vi "CAN test do RIO 2.vi"() -> ()   [LabVIEW 2014]
doc: "This example demonstrates frame streaming output using an NI-Embedded CAN for RIO interface. \n\nThis example can run against any input example, assuming you have a properly terminated CAN cable connected to two CAN ports."
uses:
  <vilib>/RioEmbeddedCAN/RioEmbeddedCAN.llb/CANFrameControl.ctl
  <vilib>/Platform/TimedLoop/XDataNode/timing_clust.ctl
  <vilib>/Platform/TimedLoop/XDataNode/nitl_modes.ctl
  <vilib>/Platform/TimedLoop/XDataNode/wakeup.ctl
  <vilib>/Platform/TimedLoop/XDataNode/XDataNode.xnode
  <vilib>/Platform/TimedLoop/XDataNode/XDNodeRunTimeDep.lvlib
  <resource>/objmgr/RioEmbeddedCANInterface.rc
  <vilib>/Utility/Variable/NI_VariableUtilities.lvlib
  Data Communication/Network Streams/Simple Network Streams/support/Network Stream Command.ctl
  <vilib>/RioEmbeddedCAN/RioEmbeddedCAN.llb/CANWaitTransmitComplete.vi
panel:
  out "okres":dbl
  out "value":T1 {"type" items=["CAN Data", "CAN Remote"]; "identifier" format="%.0x"}
  in  "stop 3":bool
  out "ilosc mesag 2":dbl
  out "Frames 3":string[][](table) caption="Frames"
  out "Numeric 2":i32
  in  "Number of Frames to Display 3":i32=15
  in  "stop 5":bool
  out "data string":string
  in  "stop 4":bool
  out "appended array":string[](array[string])
  out "ilosc mesag":dbl
  out "Numeric":i32
  in  "stop 2":bool
  out "Waveform Chart 5":cluster{"mean":dbl, "output 3":u16}(graph)
  out "Waveform Chart 2":cluster{"rms value":dbl, "output 2":dbl}(graph)
  in  "odczyt 2":bool=TRUE
  out "Frames 2":string[][](table) caption="Frames"
  in  "Number of Frames to Display 2":i32=15
  in  "Hexadecimal? 2":bool
  out "error out":errorcluster
  out "x != y?":bool
  out "(hi.lo)":u16
  out "x .or. y?":bool
  out "data":T1[](array[typedef]) {"type" items=["CAN Data", "CAN Remote"]; "identifier" format="%.0x"}
  in  "stop":bool
  out "Variable2":bool
  in  "CAN frame 2":T1={"identifier"=2, "extended?"=FALSE, "type"=0, "payload"=[1, 2, 3, 4, 5, 6, 7, 8]} {"type" items=["CAN Data", "CAN Remote"]; "identifier" format="%.0x"}
  in  "Stop Button":bool
  in  "Write":bool
  in  "CAN frame":T1={"identifier"=2, "extended?"=FALSE, "type"=0, "payload"=[1, 2, 3, 4, 5, 6, 7, 8]} {"type" items=["CAN Data", "CAN Remote"]; "identifier" format="%.0x"}
  in  "receive queue size":u32=50
  in  "baud rate":u32=500000
  in  "interface index":u32
  # "Overview: Demonstrates frame streaming output using an NI-Embedded CAN for RIO interface.\nInstructions: Run the VI."
  # "See VI Info <Ctrl+I> for more information on how to use this example"
  # "Interface Configuration"
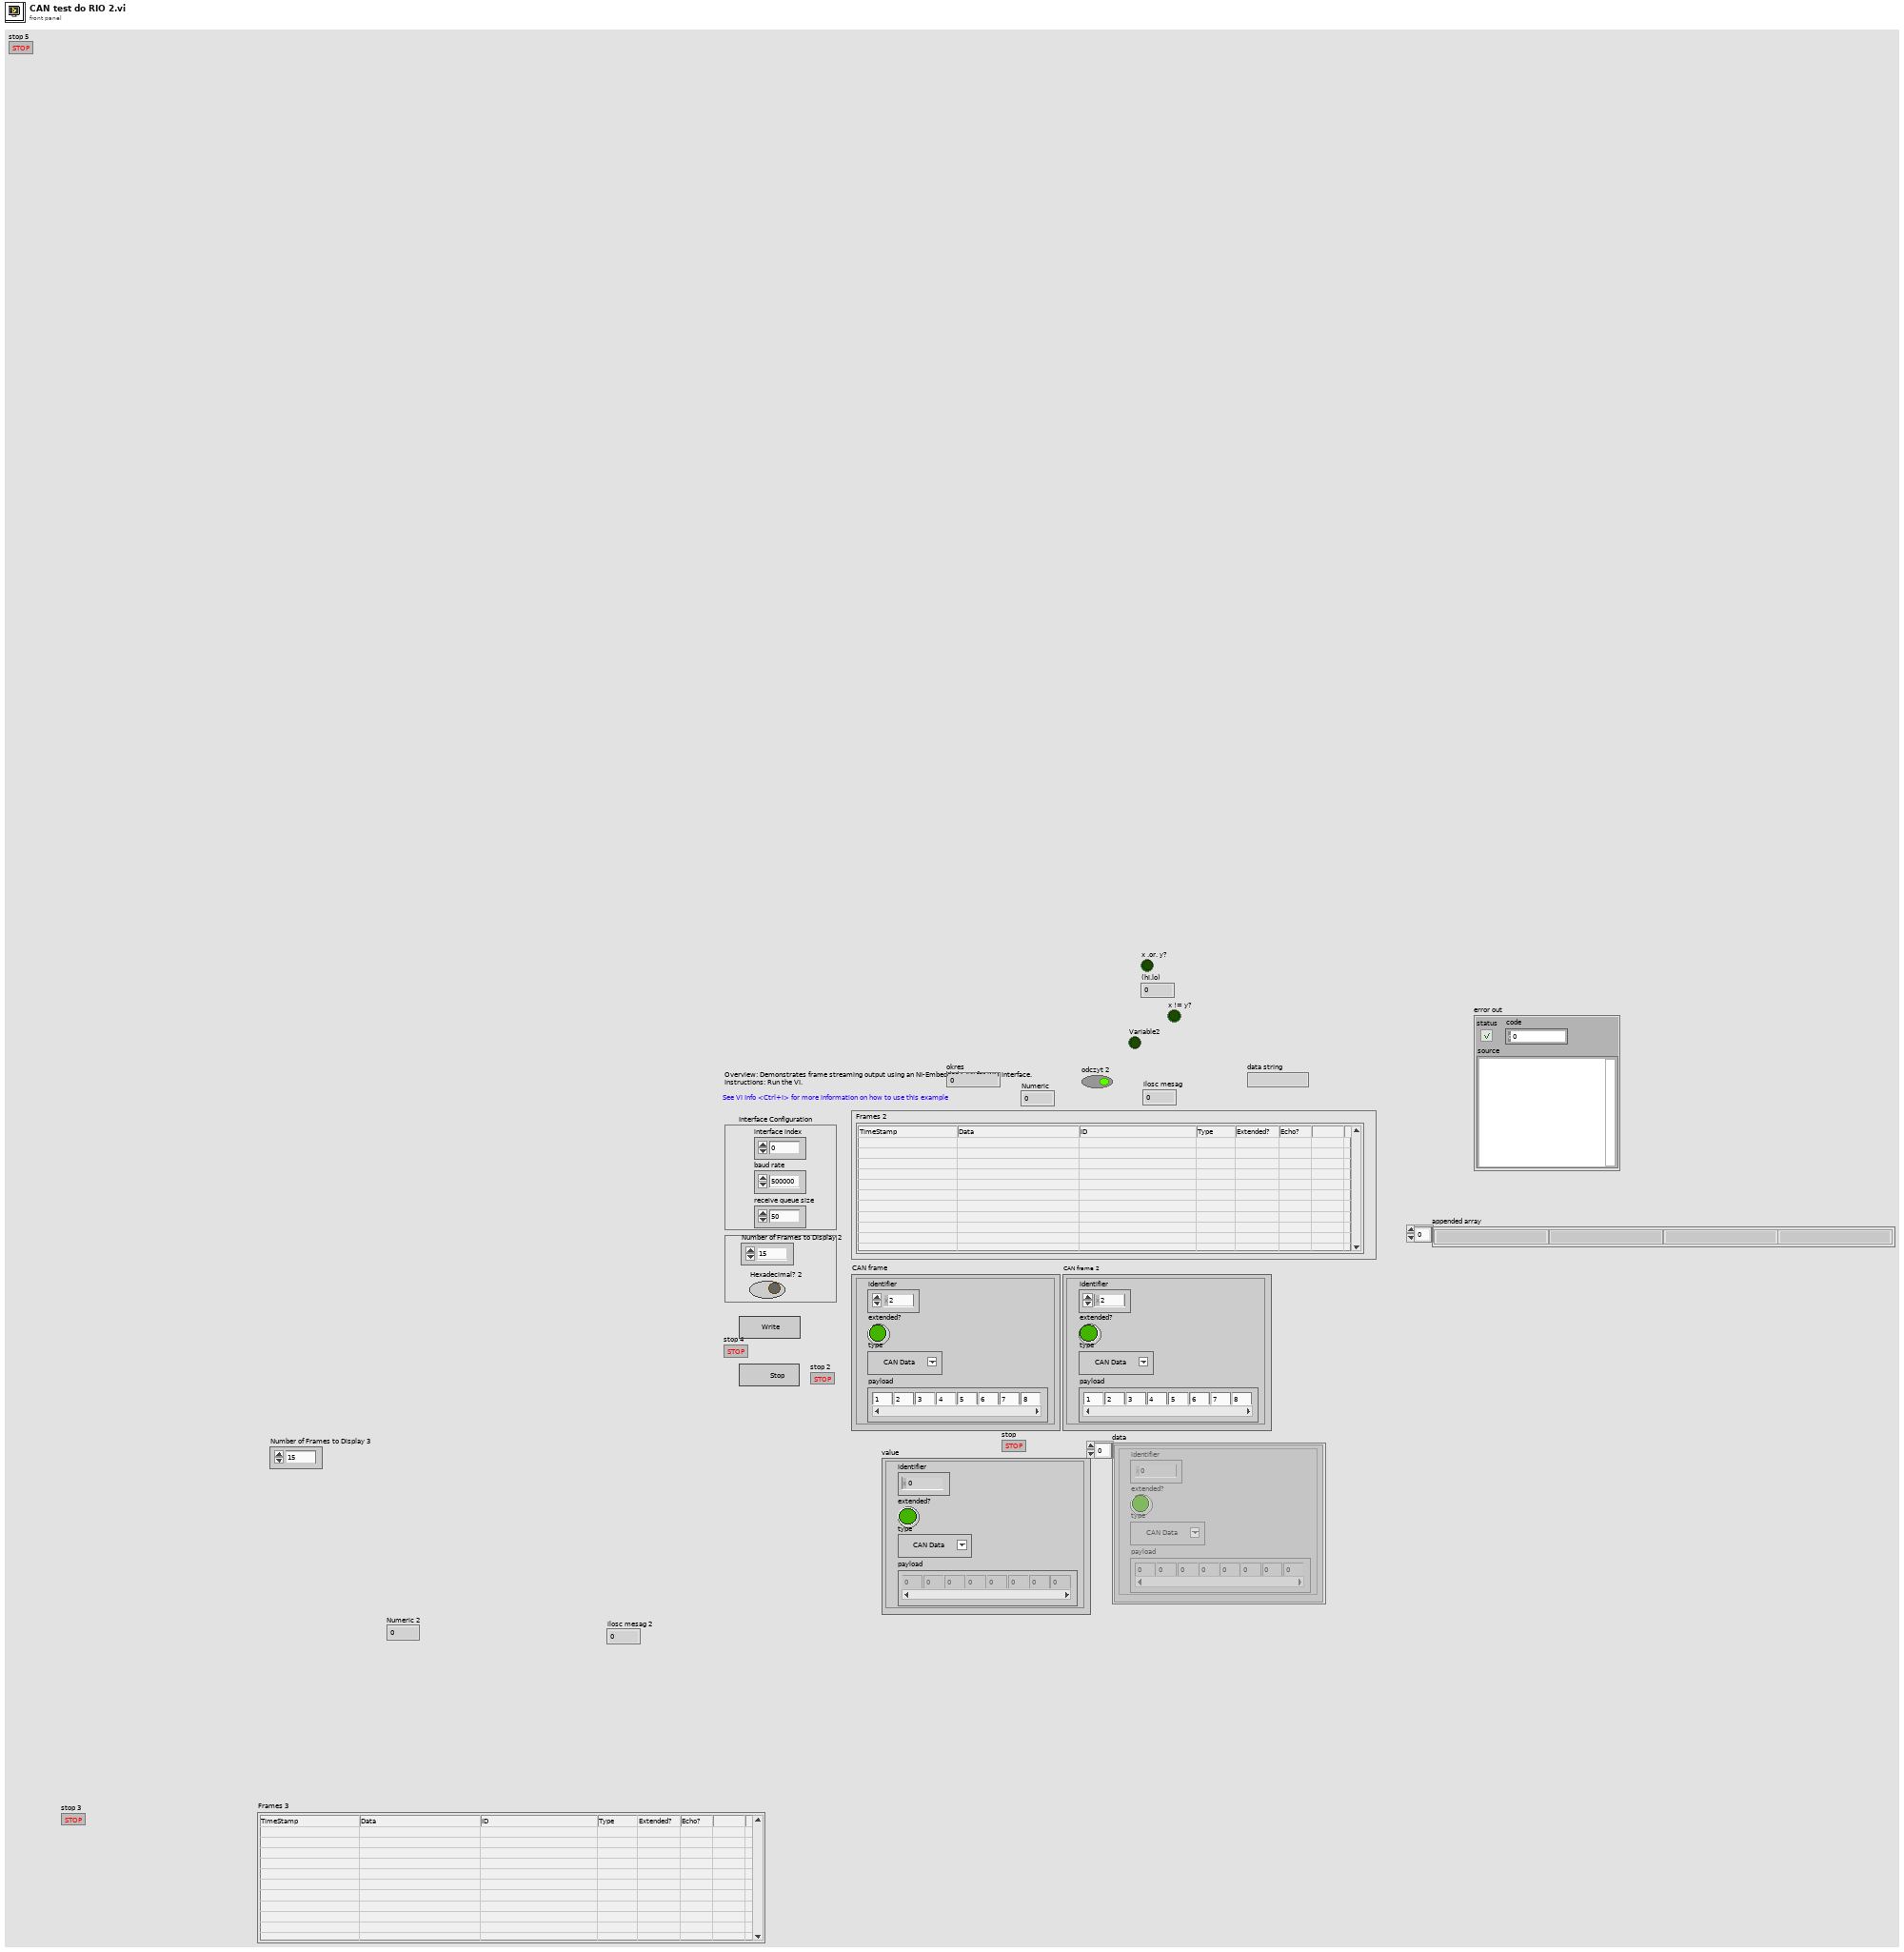
[diagram p1: front panel]
types:
  T1 = typedef "CANFrameControl.ctl" = cluster{"identifier":u32, "extended?":bool, "type":u8, "payload":u8[]}
  T2 = typedef "XDNodeRunTimeDep.lvlib/timing_clust.ctl" = cluster{"Expected End [f-1]":u64, "Actual End [f-1]":u64, "Finished Late? [f-1]":bool, "Expected End [i-1]":u64, "Actual End [i-1]":u64, "Finished Late? [i-1]":bool, "Expected Start [i]":u64, "Actual Start [i]":u64, "Expected Start [f]":u64, "Actual Start [f]":u64, "Source Name":string, "Structure Name":string, "Period":i64, "Deadline":i64, "Offset":i64, "Start":i64, "Priority":i32, "Timeout":i32, "Mode":T3, "Wakeup Reason":T4, "Error":errorcluster, "Source Type":string, "Secondary Source Type":string, "Global End Time":u64, "Global Start Time":u64, "Frame Duration":u64, "Iteration Duration":u64, "Assigned CPU":i32, "I/O Scan Engine Mode":u32}
  T3 = typedef "XDNodeRunTimeDep.lvlib/nitl_modes.ctl" = enum32{"No Change", "Process missed periods, maintain original phase", "Discard missed periods, maintain original phase", "Process missed periods, ignore original phase", "Discard missed periods, ignore original phase"}
  T4 = typedef "XDNodeRunTimeDep.lvlib/wakeup.ctl" = enum32{"Normal", "Aborted", "Asynchronous wakeup", "Timing source error", "Timed loop error", "Timeout"}
  T5 = typedef "Network Stream Command.ctl" = cluster{"Message":string, "Message Data":variant}
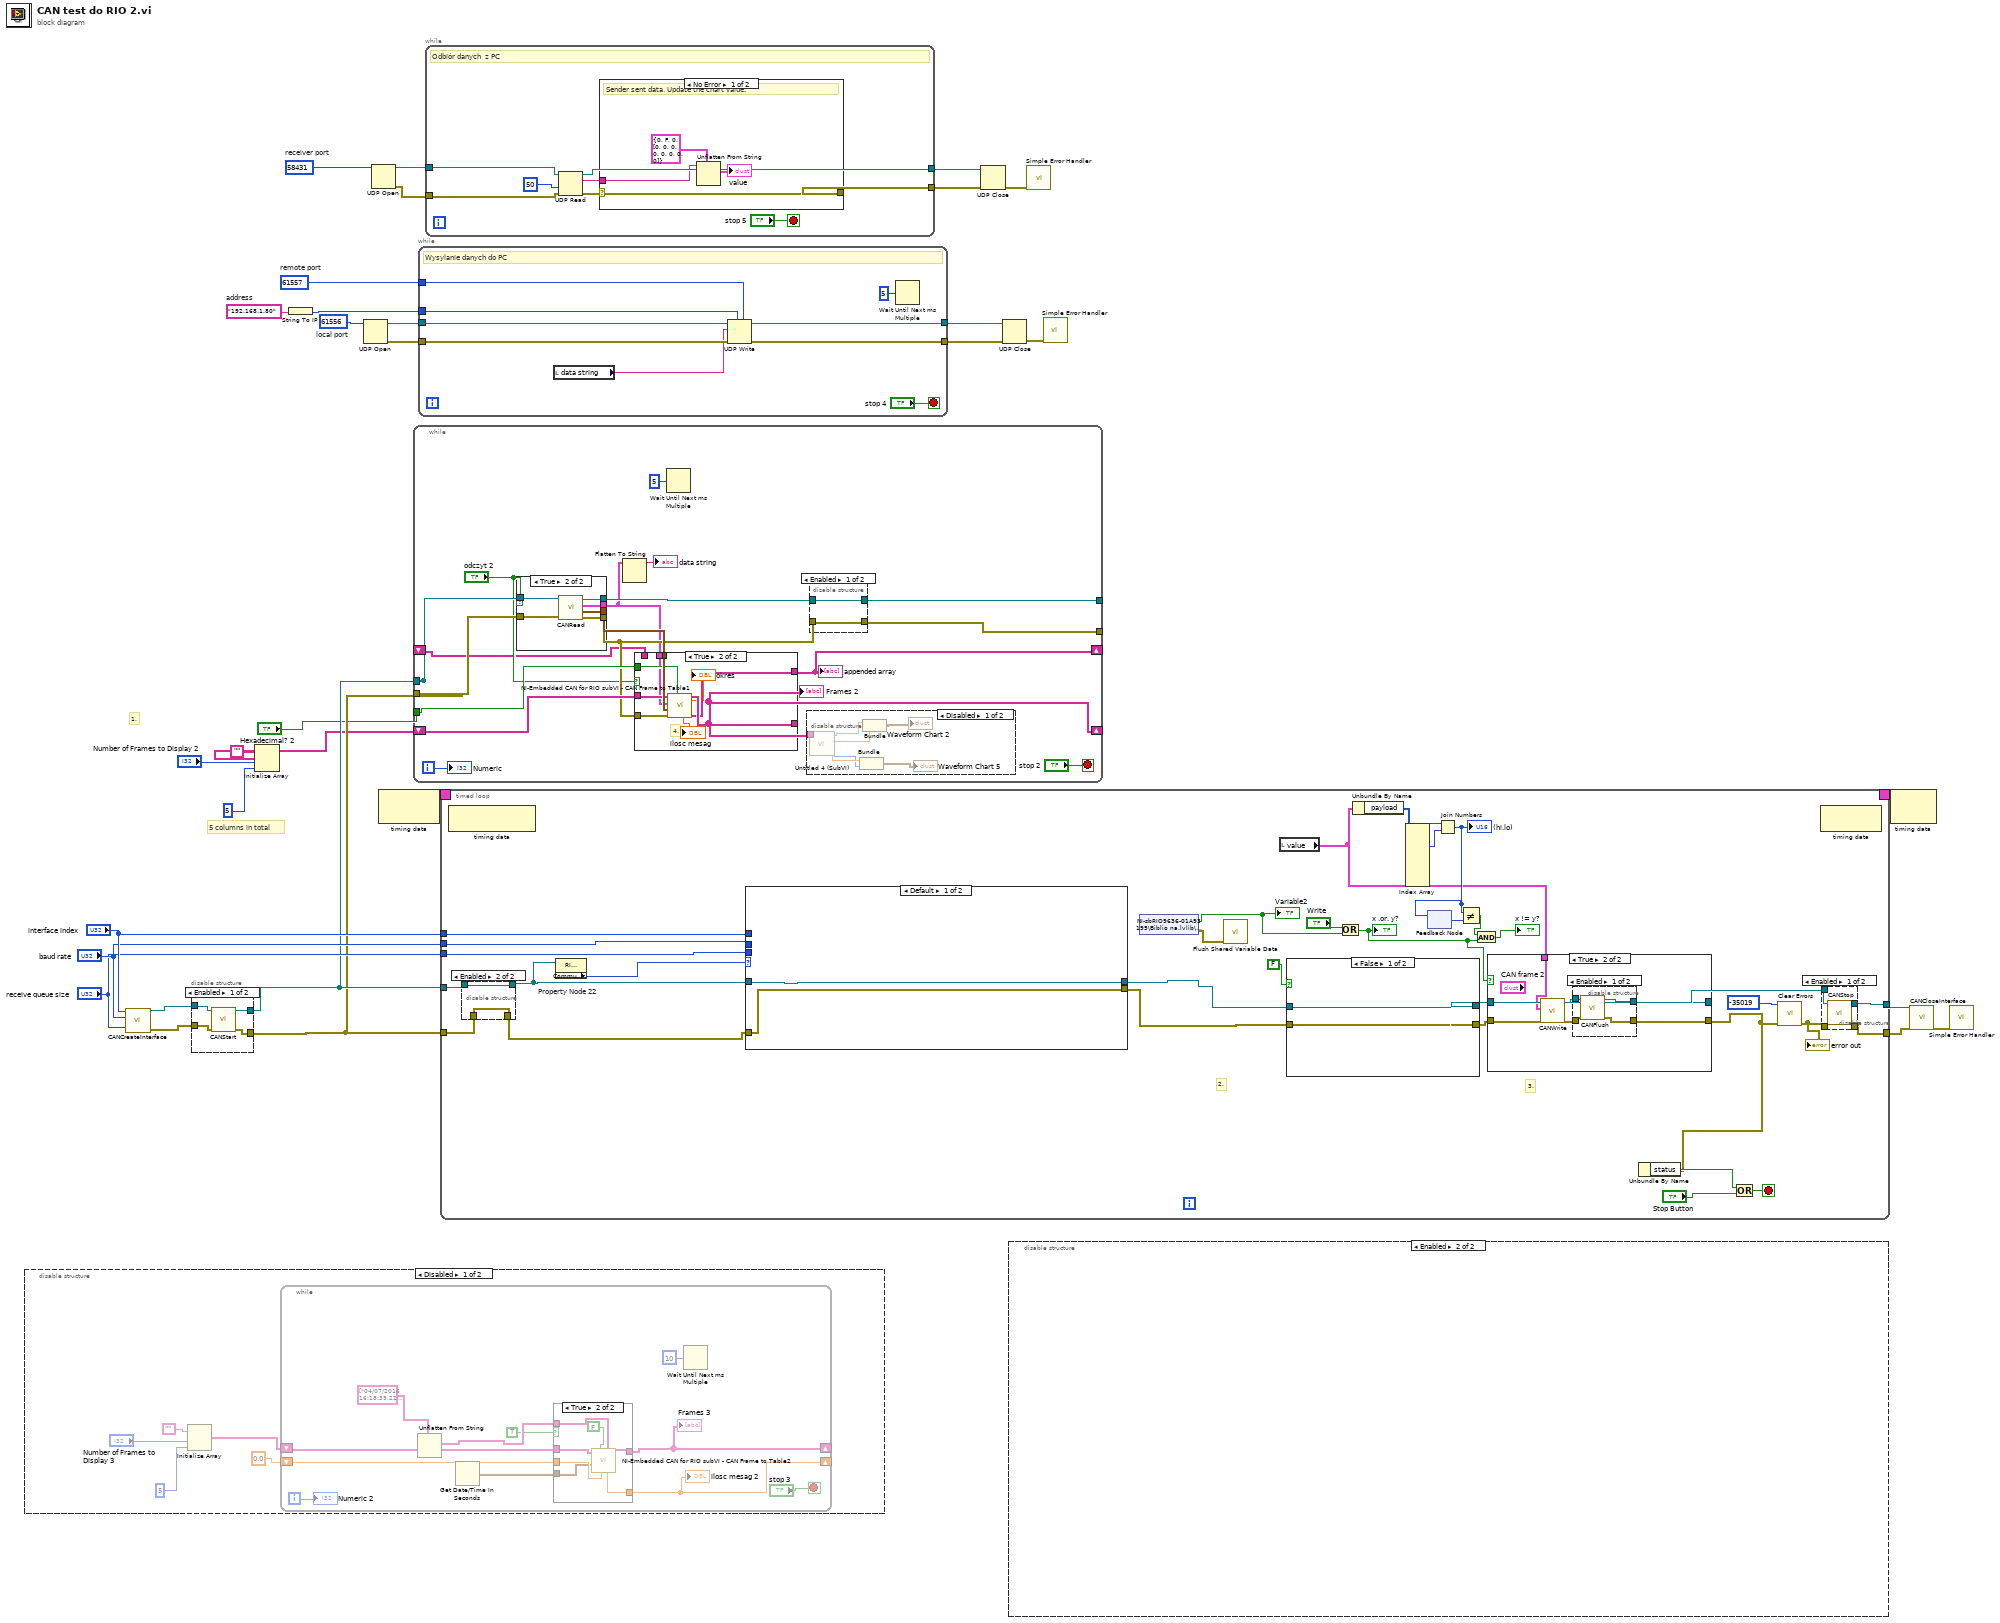
[diagram p0: block diagram]
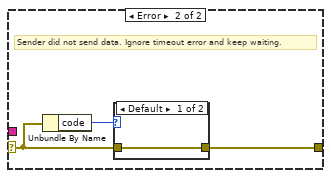
[diagram p4: hidden frame]
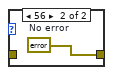
[diagram p5: hidden frame]
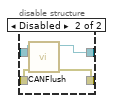
[diagram p8: hidden frame]
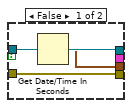
[diagram p9: hidden frame]
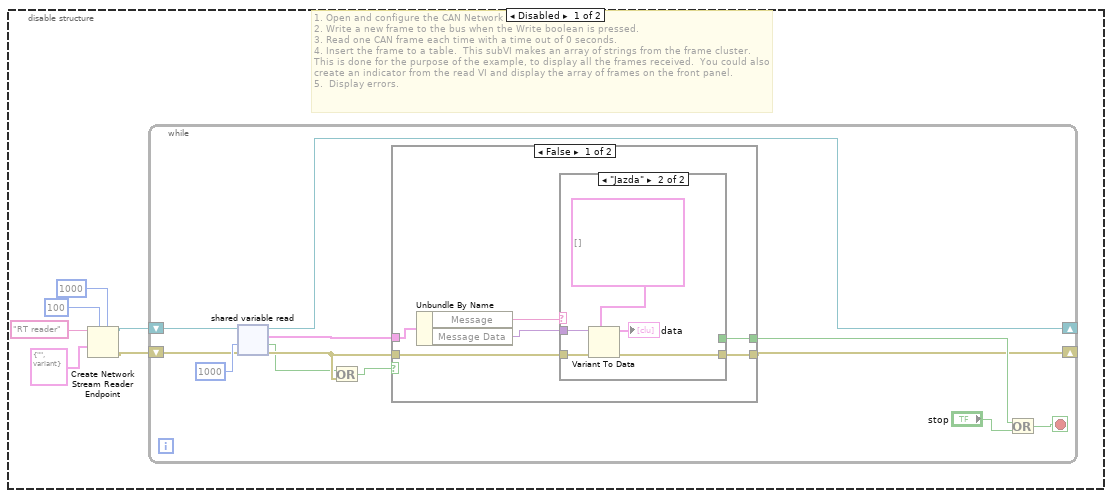
[diagram p11: hidden frame]
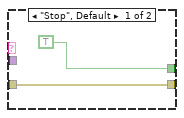
[diagram p12: hidden frame]
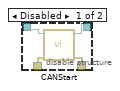
[diagram p14: hidden frame]
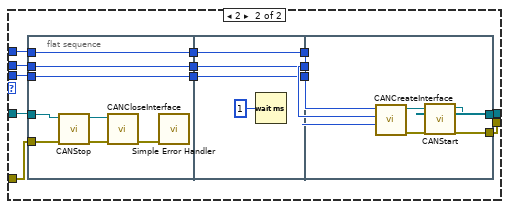
[diagram p16: hidden frame]
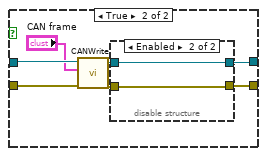
[diagram p19: hidden frame]
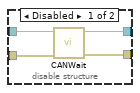
[diagram p20: hidden frame]
diagram:
  w6 = u16 58431  # receiver port
  w7 = u16 61557  # remote port
  w15 = u16 61556  # local port
  w14 = "192.168.1.80"  # address
  # "5 columns in total"
  # "1."
  n1 = disable-structure shown="Disabled" {
    frame Disabled {
      n2 = Initialize Array("" ("Empty String Constant"), "Number of Frames to Display 3", 5 ("dimension size")) -> (w33:string[][])
      n3 = while {
        shift-right: [w44] -> _
        shift-left: w33 -> [w47]
        shift-right: [w45] -> _
        shift-left: 0.0 ("Numeric") -> [w46]
        i -> [w39]
        stop <- "stop 3" stop-if-true
        n4 = Unflatten From String(type=string[] ["04/07/2016 16:18:39.223313", " 17\t 17\t 17\t 17\t 17\t 17\t 17\t 17\n", "1", "CAN Data", "No"] ("appended array")) -> (value=w42:string[])  [unwired: 4 in, 2 out]
        n5 = Get Date/Time In Seconds() -> (seconds since 1Jan1904=w43:timestamp)
        n6 = case shown="True" TRUE {
          tunnel: [w50 w57] -> w44
          tunnel: [w49 w56] -> w45
          tunnel: w47 -> [w50 w54]
          tunnel: w46 -> [w49 w55]
          tunnel: w43 -> [_ w52]
          tunnel: w42 -> [_ w51]
          frame False {
          }
          frame True {
            n7 = call "NI-Embedded CAN for RIO subVI - CAN Frame to Table2.vi"("appended array"=w51, "x"=w55, "Hexadecimal?"=FALSE, "timestamp"=w52, "Input Array"=w54) -> ("Output Array"=w57:string[][], "Numeric"=w56:dbl)  [unwired: 5 in]
          }
        }
        "ilosc mesag 2" <- w45
        "Frames 3" <- w44
        n8 = Wait Until Next ms Multiple(millisecond multiple=u32 10) -> ()  [unwired: 1 out]
        "Numeric 2" <- w39
      }
    }
    frame Enabled {
    }
  }
  n9 = call <vilib>:"CANCreateInterface.vi"("receive queue size (5)"="receive queue size", "baud rate (125000 bps)"="baud rate", "interface index"="interface index") -> ("error out"=w23:errorcluster, "interface object out"=w24:refnum<k20>)  [unwired: 7 in]
  n10 = disable-structure shown="Enabled" {
    disable-tunnel: w24 -> [w61 w63]
    disable-tunnel: [w60 w63] -> w22
    disable-tunnel: w23 -> [w59 w62]
    disable-tunnel: [w58 w62] -> w21
    frame Enabled {
      n11 = call <vilib>:"CANStart.vi"("error in (no error)"=w59, "interface object in"=w61) -> ("error out"=w58:errorcluster, "interface object out"=w60:refnum<k20>)  [unwired: 8 in]
    }
    frame Disabled {
    }
  }
  n12 = Initialize Array("" ("Empty String Constant"), "Number of Frames to Display 2", 5 ("dimension size")) -> (w17:string[][])
  n13 = String To IP(1:w14) -> (0:w8:u32)
  n14 = UDP Open(11:w15) -> (port=w12:refnum<k16>, 0:w11:errorcluster)  [unwired: 4 in, 1 out]
  n15 = UDP Open(11:w6) -> (port=w4:refnum<k16>, 0:w3:errorcluster)  [unwired: 4 in, 1 out]
  n16 = node-c288 ("Input Node")() -> (w32:T2)  [unwired: 1 in]
  n17 = while {
    tunnel: [w79] -> _
    tunnel: w22 -> [w79]
    tunnel: w21 -> [w78]
    shift-right: [w69] -> _
    shift-left: w17 -> [w75]
    tunnel: "Hexadecimal? 2" -> [w80]
    tunnel: [w77] -> _
    tunnel: [w76] -> _
    shift-right: [w67] -> _
    shift-left: _ -> [w68]
    i -> [w70]
    stop <- "stop 2" stop-if-true
    n18 = case shown="True" "odczyt 2" {
      tunnel: w79 -> [w107 w114]
      tunnel: w78 -> [w108 w113]
      tunnel: [w106 w112] -> w81
      tunnel: [w108 w111] -> w72
      tunnel: [_ w110] -> w65
      tunnel: [w107 w109] -> w73
      frame False {
        n19 = Get Date/Time In Seconds() -> (seconds since 1Jan1904=w106:timestamp)
      }
      frame True {
        n20 = call <vilib>:"CANRead.vi"("error in (no error)"=w113, "interface object in"=w114) -> ("error out"=w111:errorcluster, "timestamp"=w112:timestamp, "CAN frame"=w110:T1, "interface object out"=w109:refnum<k20>)  [unwired: 6 in]
      }
    }
    n21 = Flatten To String(anything=w65) -> (data string=→"data string":string)  [unwired: 3 in, 2 out]
    n22 = case shown="True" "odczyt 2" {
      tunnel: w81 -> [_ w99]
      tunnel: w80 -> [_ w98]
      tunnel: w75 -> [w90 w97]
      tunnel: [w90 w96] -> w69
      tunnel: w72 -> [_ w95]
      tunnel: w65 -> [_ w94]
      tunnel: [w89 w93] -> w67
      tunnel: w68 -> [w89 _]
      frame False {
      }
      frame True {
        # "4."
        n23 = call "NI-Embedded CAN for RIO subVI - CAN Frame to Table1.vi"("Hexadecimal?"=w98, "error in (no error)"=w95, "timestamp"=w99, "CAN frame"=w94, "Input Array"=w97) -> ("appended array"=w93:string[], "Output Array"=w96:string[][], "ilosc mesagy"=→"ilosc mesag":dbl, "okres 100"=→"okres":dbl)  [unwired: 2 in, 1 out]
      }
    }
    "Frames 2" <- w69
    "appended array" <- w67
    n24 = Wait Until Next ms Multiple(millisecond multiple=u32 5) -> ()  [unwired: 1 out]
    n25 = disable-structure shown="Disabled" {
      disable-tunnel: w69 -> [w82 _]
      frame Disabled {
        n26 = call "Untitled 4 (SubVI).vi"("Output Array"=w82) -> ("mean"=w88:dbl, "output 3"=w87:u16, "output 2"=w85:dbl, "rms value"=w86:dbl)  [unwired: 4 in, 3 out]
        n27 = Bundle("mean"=w88, "output 3"=w87) -> (→"Waveform Chart 5":cluster{"mean":dbl, "output 3":u16})  [unwired: 1 in]
        n28 = Bundle("rms value"=w86, "output 2"=w85) -> (→"Waveform Chart 2":cluster{"rms value":dbl, "output 2":dbl})  [unwired: 1 in]
      }
      frame Enabled {
      }
    }
    n29 = disable-structure shown="Enabled" {
      disable-tunnel: [w101 w103] -> w76
      disable-tunnel: [w100 w102] -> w77
      disable-tunnel: w72 -> [w100 w104]
      disable-tunnel: w73 -> [w101 w105]
      frame Enabled {
      }
      frame Disabled {
        n30 = call <vilib>:"CANFlush.vi"("error in (no error)"=w104, "interface object in"=w105) -> ("error out"=w102:errorcluster, "interface object out"=w103:refnum<k20>)  [unwired: 8 in]
      }
    }
    "Numeric" <- w70
  }
  n31 = while {
    tunnel: w12 -> [w123]
    tunnel: w11 -> [w122]
    tunnel: [w120] -> w10
    tunnel: [w119] -> w9
    tunnel: w8 -> [w118]
    tunnel: w7 -> [w117]
    stop <- "stop 4" stop-if-true
    # "Wysylanie danych do PC"
    n32 = local read "data string"() -> (w116:string)
    n33 = UDP Write(address=w118, port or service name=w117, connection ID=w123, data in=w116, 8:w122) -> (error out=w119:errorcluster, 3:w120:refnum<k16>)  [unwired: 1 in]
    n34 = Wait Until Next ms Multiple(millisecond multiple=u32 5) -> ()  [unwired: 1 out]
  }
  n35 = while {
    tunnel: w4 -> [w128]
    tunnel: w3 -> [w127]
    tunnel: [w126] -> w2
    tunnel: [w124] -> w1
    stop <- "stop 5" stop-if-true
    # "Odbiór danych  z PC"
    n36 = UDP Read(connection ID=w128, timeout ms (25000)=50, 8:w127) -> (data out=w130:string, error out=w129:errorcluster, 3:w124:refnum<k16>)  [unwired: 3 out]
    n37 = case shown="No Error" w129 {
      selector: w129 -> [w135 w137]
      tunnel: w130 -> [w133 _]
      tunnel: [w135 w136] -> w126
      frame No Error {
        # "Sender sent data. Update the chart value."
        n38 = Unflatten From String(type=T1 {"identifier"=0, "extended?"=FALSE, "type"=0, "payload"=[0, 0, 0, 0, 0, 0, 0, 0]} ("CAN frame"), binary string=w133) -> (value=→"value":T1)  [unwired: 3 in, 2 out]
      }
      frame Error {
        # "Sender did not send data. Ignore timeout error and keep waiting."
        n39 = Unbundle By Name(w137) -> ("code"=w138:i32)
        n40 = case shown="Default" w138 {
          tunnel: w137 -> [w139 _]
          tunnel: [w139 w140] -> w136
          frame Default {
          }
          frame 56 {
            w140 = errorcluster {"status"=FALSE, "code"=0, "source"=""}  # No error
          }
        }
      }
    }
  }
  n41 = timed-loop "Timed Loop" {
    timing: w32 -> [_]
    timing-out: [_] -> w31
    tunnel: w22 -> [w149]
    tunnel: w21 -> [w148]
    tunnel: [w152] -> w29
    tunnel: [w150] -> w28
    tunnel: "interface index" -> [w157]
    tunnel: "baud rate" -> [w156]
    tunnel: "receive queue size" -> [w155]
    stop <- w172 stop-if-true
    # "3."
    # "2."
    n42 = node-c288 ("Output Node")() -> ()  [unwired: 1 in, 1 out]
    n43 = disable-structure shown="Enabled" {
      disable-tunnel: w149 -> [w177 w178]
      disable-tunnel: [w176 w178] -> w145
      disable-tunnel: w148 -> [w175 w179]
      disable-tunnel: [w174 w179] -> w147
      frame Disabled {
        n44 = call <vilib>:"CANStart.vi"("error in (no error)"=w175, "interface object in"=w177) -> ("error out"=w174:errorcluster, "interface object out"=w176:refnum<k20>)  [unwired: 8 in]
      }
      frame Enabled {
      }
    }
    n45 = property on="Property Node 22" class="RIOEmbeddedCAN Interface"(reference=w145) -> ("Communication State"=w144:u32)  [unwired: 1 in, 2 out]
    n46 = case shown="Default" w144 {
      tunnel: [w186 w200] -> w158
      tunnel: w145 -> [w187 w196]
      tunnel: [w187 w194] -> w146
      tunnel: w157 -> [_ w199]
      tunnel: w156 -> [_ w198]
      tunnel: w155 -> [_ w197]
      tunnel: w147 -> [w186 w195]
      frame Default {
      }
      frame 2 {
        n47 = flat-sequence {
          tunnel: w196 -> [w204]
          tunnel: w197 -> [w206]
          tunnel: w198 -> [w207]
          tunnel: w199 -> [w208]
          tunnel: [w208] -> w193
          tunnel: [w207] -> w191
          tunnel: [w206] -> w189
          tunnel: w195 -> [w201]
          tunnel: w193 -> [w212]
          tunnel: [w212] -> w192
          tunnel: w191 -> [w211]
          tunnel: [w211] -> w190
          tunnel: w189 -> [w210]
          tunnel: [w210] -> w188
          tunnel: [w214] -> w200
          tunnel: [w215] -> w194
          tunnel: w192 -> [w219]
          tunnel: w190 -> [w218]
          tunnel: w188 -> [w217]
          frame #0 {
            n48 = call <vilib>:"CANStop.vi"("error in (no error)"=w201, "interface object in"=w204) -> ("error out"=w202:errorcluster, "interface object out"=w203:refnum<k20>)  [unwired: 8 in]
            n49 = call <vilib>:"CANCloseInterface.vi"("error in (no error)"=w202, "interface object in"=w203) -> ("error out"=w205:errorcluster)  [unwired: 9 in]
            n50 = call <vilib>:"Simple Error Handler.vi"("error in (no error)"=w205) -> ()  [unwired: 4 in, 5 out]
          }
          frame #1 {
            n51 = Wait (ms)(milliseconds to wait=u32 1) -> ()  [unwired: 1 out]
          }
          frame #2 {
            n52 = call <vilib>:"CANCreateInterface.vi"("receive queue size (5)"=w217, "baud rate (125000 bps)"=w218, "interface index"=w219) -> ("error out"=w213:errorcluster, "interface object out"=w216:refnum<k20>)  [unwired: 7 in]
            n53 = call <vilib>:"CANStart.vi"("error in (no error)"=w213, "interface object in"=w216) -> ("error out"=w214:errorcluster, "interface object out"=w215:refnum<k20>)  [unwired: 8 in]
          }
        }
      }
    }
    n54 = shared-variable "NI-sbRIO9636-01A93195\\Biblio na.lvlib\\status"() -> (w169:bool, error out=w170:errorcluster)  [unwired: 1 in]
    "Variable2" <- w169
    n55 = call <vilib>:"Flush Shared Variable Data.vi"("error in (no error)"=w170) -> ()  [unwired: 10 in, 1 out]
    n56 = local read "value"() -> (w141:T1)
    n57 = case shown="False" FALSE {
      tunnel: w146 -> [w235 w243]
      tunnel: w158 -> [w236 w242]
      tunnel: [w235 w240] -> w143
      tunnel: [w236 w239] -> w167
      frame False {
      }
      frame True {
        n58 = call <vilib>:"CANWrite.vi"("error in (no error)"=w242, "CAN frame"="CAN frame", "interface object in"=w243) -> ("error out"=w238:errorcluster, "interface object out"=w241:refnum<k20>)  [unwired: 7 in]
        n59 = disable-structure shown="Enabled" {
          disable-tunnel: w241 -> [w247 w249]
          disable-tunnel: [w246 w249] -> w240
          disable-tunnel: [w245 w248] -> w239
          disable-tunnel: w238 -> [w244 w248]
          frame Disabled {
            n60 = call-poly <vilib>:"CANWait.vi"("error in (no error)"=w244, "interface object in"=w247) -> ("error out"=w245:errorcluster, "interface object out"=w246:refnum<k20>)  [unwired: 8 in]
          }
          frame Enabled {
          }
        }
      }
    }
    n61 = Or(x="Write", y=w169) -> (x .or. y?=w154:bool)
    "x .or. y?" <- w154
    n62 = Unbundle By Name(w141) -> ("payload"=w165:u8[])
    n63 = Index Array(array=w165) -> (element #1=w163:u8, element #2=w164:u8)  [unwired: 8 in, 6 out]
    n64 = feedback #1() -> (w161:u16)  [unwired: 1 in]
    n65 = Join Numbers(hi=w163, lo=w164) -> ((hi.lo)=w162:u16)
    "(hi.lo)" <- w162
    n66 = feedback-in #1(w162) -> ()
    n67 = Not Equal?(x=w162, y=w161) -> (x != y?=w160:bool)
    n68 = And(x=w160, y=w154) -> (x .and. y?=→"x != y?":bool)
    n69 = case shown="True" w154 {
      tunnel: w167 -> [w221 w224]
      tunnel: [w220 w223] -> _
      tunnel: [w221 w222] -> w142
      tunnel: w143 -> [w220 w225]
      tunnel: w141 -> [_ w226]
      frame False {
      }
      frame True {
        n70 = call <vilib>:"CANWrite.vi"("error in (no error)"=w224, "CAN frame"=w226, "interface object in"=w225) -> ("error out"=w227:errorcluster, "interface object out"=w228:refnum<k20>)  [unwired: 7 in]
        n71 = disable-structure shown="Enabled" {
          disable-tunnel: w228 -> [w232 w234]
          disable-tunnel: w227 -> [w231 w233]
          disable-tunnel: [w230 w234] -> w223
          disable-tunnel: [w229 w233] -> w222
          frame Enabled {
            n72 = call <vilib>:"CANFlush.vi"("error in (no error)"=w231, "interface object in"=w232) -> ("error out"=w229:errorcluster, "interface object out"=w230:refnum<k20>)  [unwired: 8 in]
          }
          frame Disabled {
          }
        }
      }
    }
    n73 = Unbundle By Name(w142) -> ("status"=w173:bool)
    n74 = Or(x=w173, y="Stop Button") -> (x .or. y?=w172:bool)
    n75 = call <vilib>:"Clear Errors.vi"("error in (no error)"=w142, "specific error code to clear (0: all)"=-35019) -> ("error out"=w151:errorcluster)  [unwired: 4 in, 1 out]
    "error out" <- w151
    n76 = node-c288 ("Input Node")() -> ()  [unwired: 1 in, 1 out]
    n77 = disable-structure shown="Enabled" {
      disable-tunnel: w143 -> [w183 w185]
      disable-tunnel: [w182 w185] -> w152
      disable-tunnel: w151 -> [w181 w184]
      disable-tunnel: [w180 w184] -> w150
      frame Enabled {
        n78 = call <vilib>:"CANStop.vi"("error in (no error)"=w181, "interface object in"=w183) -> ("error out"=w180:errorcluster, "interface object out"=w182:refnum<k20>)  [unwired: 8 in]
      }
      frame Disabled {
      }
    }
  }
  n79 = UDP Close(connection ID=w1, 8:w2) -> (error out=w5:errorcluster)  [unwired: 1 out]
  n80 = UDP Close(connection ID=w10, 8:w9) -> (error out=w13:errorcluster)  [unwired: 1 out]
  n81 = disable-structure shown="Enabled" {
    frame Disabled {
      # "1. Open and configure the CAN Network Interface.\n2. Write a new frame to the bus when the Write boolean is pressed.\n3. Read one CAN frame each time with a time out of 0 seconds.\n4. Insert the frame to a table.  This subVI makes an array of strings from the frame cluster.  This is done for the purpose of the example, to display all the frames received.  You could also create an indicator from the read VI and display the array of frames on the front panel. \n5.  Display errors."
      n82 = Create Network Stream Reader Endpoint(5:1000 ("timeout in ms (-1)"), 7:100 ("reader buffer size"), 9:T5 {"Message"="", "Message Data"=variant} ("Message Cluster"), 11:"RT reader" ("reader url")) -> (0:w253:errorcluster, 3:w254:refnum<k21>)  [unwired: 3 in]
      n83 = while {
        shift-right: [w258] -> _
        shift-left: w254 -> [w268]
        shift-right: [w259] -> _
        shift-left: w253 -> [w267]
        stop <- w261 stop-if-true
        n84 = shared-variable-read(w268, w267, 1000 ("timeout ms")) -> (w258:refnum<k21>, w264:errorcluster, w263:bool, w266:T5)
        n85 = Or(x=w263, y=w264) -> (x .or. y?=w265:bool)
        n86 = case shown="False" w265 {
          tunnel: w264 -> [w275 w283]
          tunnel: [w274 w283] -> w259
          tunnel: [w273 _] -> w260
          tunnel: w266 -> [w272 _]
          frame False {
            n87 = Unbundle By Name(w272) -> ("Message"=w271:string, "Message Data"=w270:variant)
            n88 = case shown="\"Jazda\"" w271 {
              tunnel: w275 -> [w277 w282]
              tunnel: [w277 w281] -> w274
              tunnel: [TRUE _] -> w273
              tunnel: w270 -> [_ w280]
              frame "Stop", Default {
              }
              frame "Jazda" {
                n89 = Variant To Data(error in=w282, type=T1[] [], Variant=w280) -> (data=→"data":T1[], error out=w281:errorcluster)
              }
            }
          }
          frame True {
          }
        }
        n90 = Or(x=w260, y="stop") -> (x .or. y?=w261:bool)
      }
    }
    frame Enabled {
    }
  }
  n91 = call <vilib>:"Simple Error Handler.vi"("error in (no error)"=w5) -> ()  [unwired: 1 in, 8 out]
  n92 = call <vilib>:"Simple Error Handler.vi"("error in (no error)"=w13) -> ()  [unwired: 4 in, 5 out]
  n93 = node-c288 ("Output Node")(w31) -> ()  [unwired: 1 out]
  n94 = call <vilib>:"CANCloseInterface.vi"("error in (no error)"=w28, "interface object in"=w29) -> ("error out"=w30:errorcluster)  [unwired: 9 in]
  n95 = call <vilib>:"Simple Error Handler.vi"("error in (no error)"=w30) -> ()  [unwired: 4 in, 5 out]
